vi "Traffic Lights.vi"() -> ()   [LabVIEW 2023]
uses:
  Traffic Lights Control.ctl
panel:
  in  "?":bool
  out "Red Light":bool
  out "Yellow Light":bool
  out "Green Light":bool
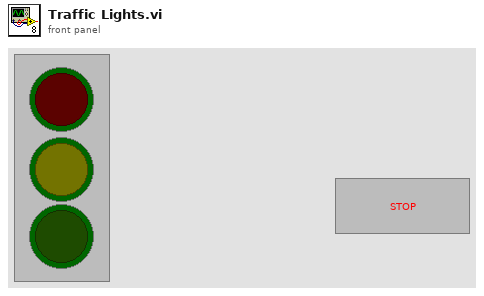
[diagram p1: front panel]
types:
  T1 = typedef "Traffic Lights Control.ctl" = enum16{"Green", "Yellow", "Red"}
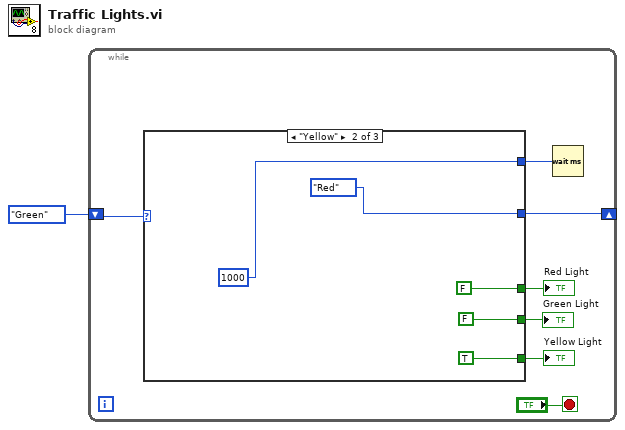
[diagram p0: block diagram]
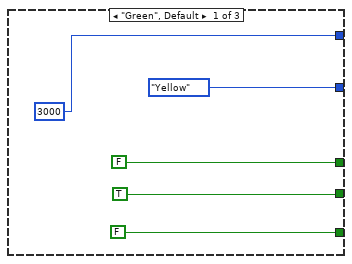
[diagram p2: hidden frame]
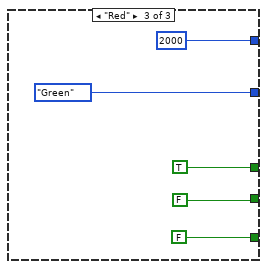
[diagram p3: hidden frame]
diagram:
  n1 = while {
    shift-right: [w7] -> _
    shift-left: Traffic_Lights_Control."Green" -> [w8]
    stop <- "?" stop-if-true
    n2 = case shown="\"Yellow\"" w8 {
      tunnel: [Traffic_Lights_Control."Yellow" Traffic_Lights_Control."Red" Traffic_Lights_Control."Green"] -> w7
      tunnel: [FALSE ("Green Light") FALSE ("Green Light") TRUE ("Green Light")] -> w5
      tunnel: [FALSE TRUE ("Green Light") FALSE ("Green Light")] -> w4
      tunnel: [TRUE ("Green Light") FALSE ("Green Light") FALSE ("Green Light")] -> w3
      tunnel: [u32 3000 ("milliseconds to wait") u32 1000 ("milliseconds to wait") u32 2000 ("milliseconds to wait")] -> w2
      frame "Green", Default {
      }
      frame "Yellow" {
      }
      frame "Red" {
      }
    }
    "Red Light" <- w5
    "Green Light" <- w3
    "Yellow Light" <- w4
    n3 = Wait (ms)(milliseconds to wait=w2) -> ()  [unwired: 1 out]
  }
